vi "Add Status Lookup Data.vi"(8 "value index":i32, 9 "terminal handle":u64, 10 "terminal address":T2, 11 "status lookup array":T1[](array[typedef]) {"terminal address" format="%.0x"; "remote terminal handle" format="%.0x"}) -> (0 "value index +1":i32, 3 "status lookup array out":T1[](array[typedef]) {"terminal address" format="%.0x"; "remote terminal handle" format="%.0x"})   [LabVIEW 2023, in "Ballard MIL-STD-1553 Engine Support.lvlib" / "Custom Device.lvlib"]
uses:
  Custom Device.lvlib
  Shared/Address.ctl
  Implementation/Rx Execution Unit/Status Terminal Lookup Data.ctl
  Implementation/Rx Execution Unit/Rx Execution Unit.lvclass
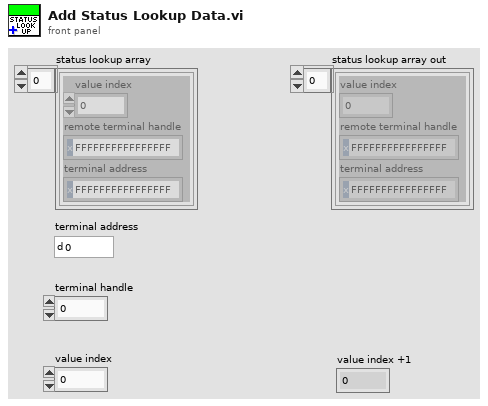
[diagram p1: front panel]
types:
  T1 = typedef "Ballard MIL-STD-1553 Engine Support.lvlib/Implementation.lvlib/Rx Execution Unit.lvclass/Status Terminal Lookup Data.ctl" = cluster{"value index":i32, "remote terminal handle":u64, "terminal address":u64}
  T2 = typedef "Address.ctl" = u16
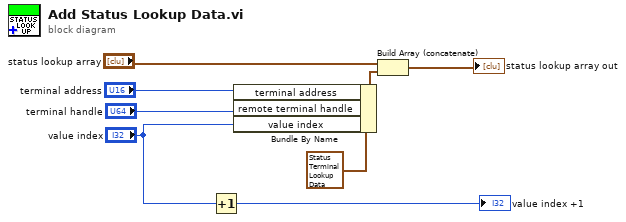
[diagram p0: block diagram]
diagram:
  n1 = Increment(x="value index") -> (x+1=→"value index +1":i32)
  n2 = Bundle By Name(cluster=T1 {"value index"=0, "remote terminal handle"=18446744073709551615, "terminal address"=18446744073709551615} ("status lookup data"), "terminal address"="terminal address", "remote terminal handle"="terminal handle", "value index"="value index") -> (w8:T1)
  n3 = Build Array (concatenate)("status lookup array", w8) -> (→"status lookup array out":T1[])
